vi "2d Gaussian array.vi"() -> (3 "Array":u8[][](array[numeric]))   [LabVIEW 2020]
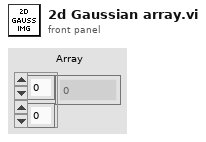
[diagram p1: front panel]
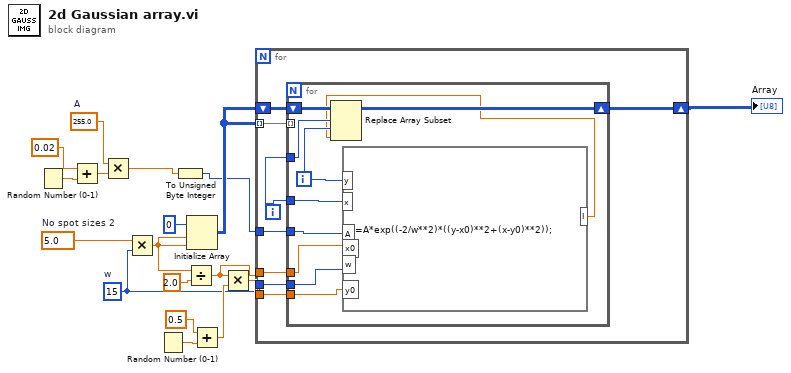
[diagram p0: block diagram]
diagram:
  w18 = 255.0  # A
  w7 = 5.0  # No spot sizes 2
  w8 = u8 15  # w
  n1 = Random Number (0-1)() -> (number: 0 to 1=w17:dbl)
  n2 = Add(x=0.02, y=w17) -> (x+y=w16:dbl)
  n3 = Multiply(x=w18, y=w16) -> (x*y=w3:dbl)
  n4 = Multiply(x=w7, y=w8) -> (x*y=w6:dbl)
  n5 = Random Number (0-1)() -> (number: 0 to 1=w11:dbl)
  n6 = To Unsigned Byte Integer(number=w3) -> (unsigned 8bit integer=w2:u8)
  n7 = Divide(x=w6, y=2.0) -> (x/y=w14:dbl)
  n8 = Initialize Array(u8 0 ("element"), w6, w6) -> (w9:u8[][])
  n9 = Add(x=0.5, y=w11) -> (x+y=w13:dbl)
  n10 = Multiply(x=w14, y=w13) -> (x*y=w15:dbl)
  n11 = for {
    tunnel: w9 -> [w26] mode=indexing
    shift-right: [w24] -> w4
    shift-left: w9 -> [w25]
    tunnel: w2 -> [w23]
    tunnel: w14 -> [w21]
    tunnel: w8 -> [w20]
    tunnel: w15 -> [w19]
    i -> [w22]
    n12 = for {
      tunnel: w26 -> [_] mode=indexing
      shift-right: [w35] -> w24
      shift-left: w25 -> [w36]
      tunnel: w22 -> [w34]
      tunnel: w23 -> [w31]
      tunnel: w22 -> [w30]
      tunnel: w21 -> [w29]
      tunnel: w20 -> [w28]
      tunnel: w19 -> [w27]
      i -> [w33]
      n13 = formula code="I=A*exp((-2/w**2)*((y-x0)**2+(x-y0)**2));"("y"=w33, "A"=w31, "x0"=w29, "x"=w30, "w"=w28, "y0"=w27) -> ("I"=w32:dbl)
      n14 = Replace Array Subset(array=w36, new element=w32, index (row)=w34, index (col)=w33) -> (w35:u8[][])
    }
  }
  "Array" <- w4
